vi "CAN loopback test.vi"() -> ()   [LabVIEW 2014]
uses:
  <vilib>/Utility/sysdir.llb/System Directory Type.ctl
  <vilib>/xnet/xnet.llb/XNET Frame CAN.ctl
  <vilib>/xnet/xnet.llb/XNET Frame Type CAN.ctl
  <vilib>/xnet/xnet.llb/XNET Create Session (Frame Input Stream).vi
  <vilib>/xnet/xnet.llb/XNET Create Session (Frame Output Stream).vi
  <vilib>/xnet/xnet.llb/XNET Write (Frame CAN).vi
  <vilib>/xnet/xnet.llb/XNET Read (Frame CAN).vi
  <resource>/objmgr/xnet.rc
panel:
  out "iteration":i32
  out "Frame Passed":bool
  in  "Suspected interface (transmitting)":refnum<k21>="CAN2"
  in  "Termination - set to On, since cables are unterminated":u32(ring)=1 items=["Off", "On"]
  in  "Receiving CAN port (known good module)":refnum<k21>="CAN1"
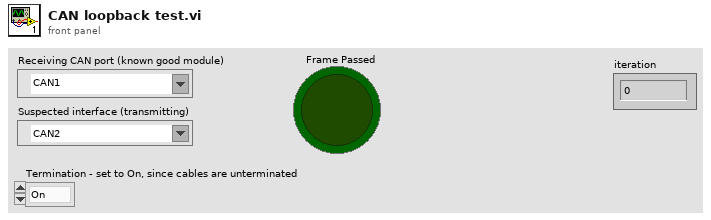
[diagram p1: front panel]
types:
  T1 = typedef "System Directory Type.ctl" = i32
  T2 = enum16{"open", "replace", "create", "open or create", "replace or create", "replace or create with confirmation"}
  T3 = typedef "XNET Frame CAN.ctl" = cluster{"timestamp":timestamp, "payload":u8[], "identifier":u32, "type":T4, "extended?":bool, "echo?":bool}
  T4 = typedef "XNET Frame Type CAN.ctl" = u8
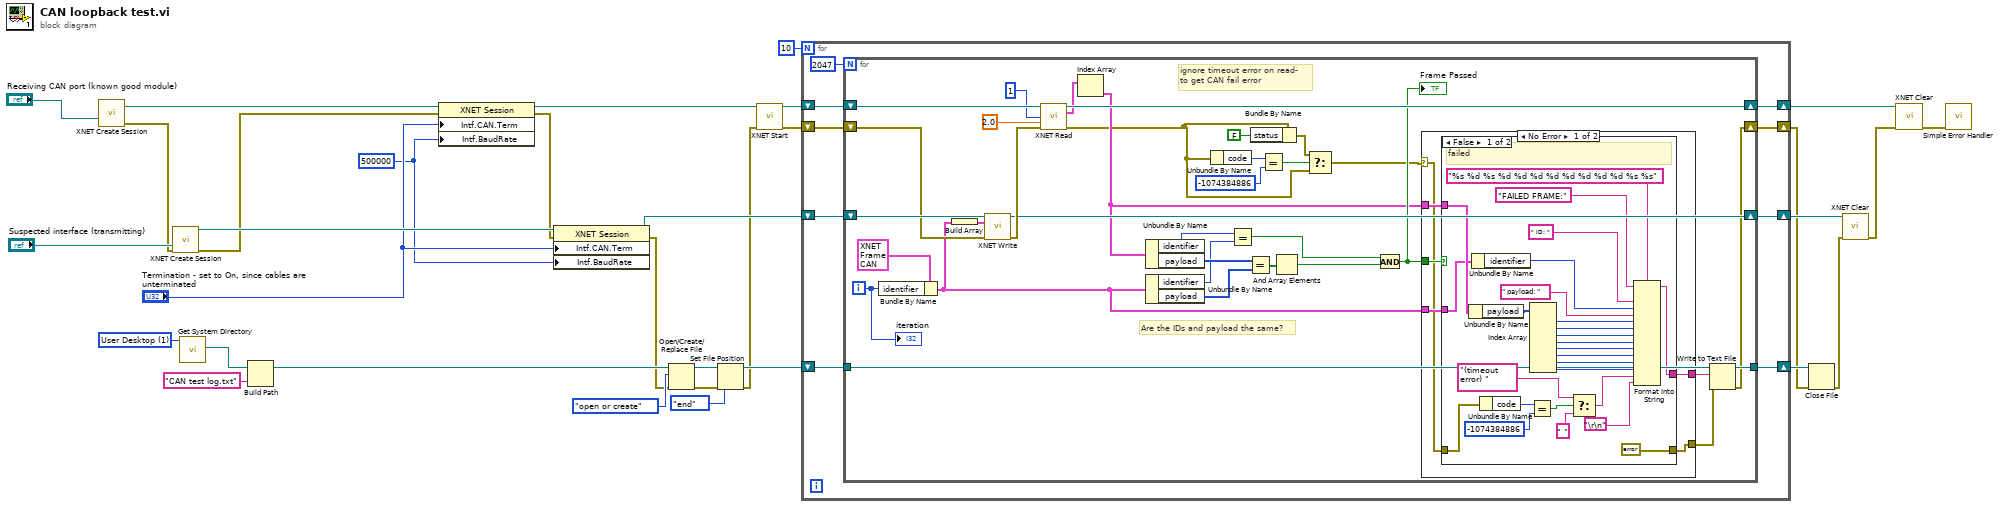
[diagram p0: block diagram]
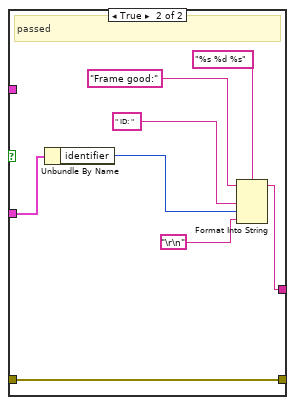
[diagram p2: hidden frame]
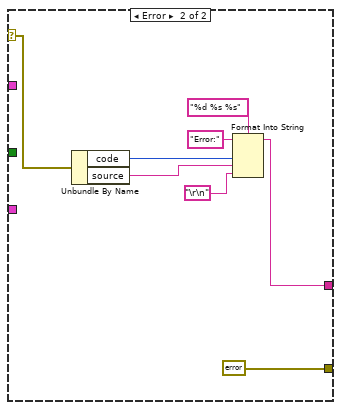
[diagram p3: hidden frame]
diagram:
  w4 = u32 500000 ("Interface:Baud Rate")
  w13 = T1 1 items=["User Home"=0, "User Desktop"=1, "User Documents"=2, "User Application Data"=3, "User Preferences"=4, "User Temporary"=5, "Public Documents"=6, "Public Application Data"=7, "Public Preferences"=8, "Public Cache"=13, "System Core Libraries"=9, "System Installed Libraries"=10, "Application Files"=11, "Boot Volume Root"=12] ("system directory type")
  n1 = call-poly <vilib>:"XNET Create Session.vi"("interface"="Receiving CAN port (known good module)") -> ("session out"=w7:refnum<k21>, "error out"=w28:errorcluster)  [unwired: 2 in, 11 out]
  n2 = call-poly <vilib>:"XNET Create Session.vi"("interface"="Suspected interface (transmitting)", "error in (no error)"=w28) -> ("session out"=w22:refnum<k21>, "error out"=w1:errorcluster)  [unwired: 1 in, 11 out]
  n3 = call <vilib>:"Get System Directory.vi"("system directory type"=w13) -> ("system directory"=w12:path)  [unwired: 10 in]
  n4 = Build Path(base path=w12, name or relative path="CAN test log.txt") -> (appended path=w11:path)
  n5 = property class="XNET Session"(reference=w7, error in=w1, "Intf.CAN.Term"="Termination - set to On, since cables are unterminated", "Intf.BaudRate"=w4) -> (reference out=w6:refnum<k21>, error out=w2:errorcluster)
  n6 = property class="XNET Session"(reference=w22, error in=w2, "Intf.CAN.Term"="Termination - set to On, since cables are unterminated", "Intf.BaudRate"=w4) -> (reference out=w31:refnum<k21>, error out=w9:errorcluster)
  n7 = Open/Create/Replace File(file path (use dialog)=w11, error in=w9, operation (0:open)=T2."open or create") -> (refnum out=w16:refnum<file>, error out=w21:errorcluster)  [unwired: 3 in, 1 out]
  n8 = Set File Position(refnum=w16, from (0:start)=enum16{"start", "end", "current"}."end", error in=w21) -> (refnum out=w15:refnum<file>, error out=w8:errorcluster)  [unwired: 1 in]
  n9 = call <vilib>:"XNET Start.vi"("session in"=w6, "error in (no error)"=w8) -> ("session out"=w27:refnum<k21>, "error out"=w29:errorcluster)  [unwired: 12 in]
  n10 = for {
    N: 10 -> [_]
    shift-right: [w38] -> w26
    shift-left: w31 -> [w41]
    shift-right: [w35] -> w19
    shift-left: w29 -> [w40]
    shift-right: [w37] -> w25
    shift-left: w27 -> [w39]
    shift-right: [w36] -> w20
    shift-left: w15 -> [w34]
    n11 = for {
      N: 2047 ("Numeric Control") -> [_]
      shift-right: [w70] -> w38
      shift-left: w41 -> [w75]
      shift-right: [w49] -> w35
      shift-left: w40 -> [w74]
      shift-right: [w69] -> w37
      shift-left: w39 -> [w72]
      tunnel: w34 -> [w52]
      tunnel: [w53] -> w36
      i -> [w62]
      # "ignore timeout error on read-\nto get CAN fail error"
      # "Are the IDs and payload the same?"
      n12 = Bundle By Name(cluster=T3 {"timestamp"=timestamp(0 s since 1904-01-01), "payload"=[0, 1, 2, 3, 4, 5, 6, 7], "identifier"=0, "type"=0, "extended?"=FALSE, "echo?"=FALSE} ("CAN frame"), "identifier"=w62) -> (w55:T3)
      n13 = Build Array(w55) -> (w61:T3[])
      n14 = call-poly <vilib>:"XNET Write.vi"("session in"=w75, "data"=w61, "error in (no error)"=w74) -> ("session out"=w70:refnum<k21>, "error out"=w73:errorcluster)  [unwired: 11 out]
      n15 = call-poly <vilib>:"XNET Read.vi"("session in"=w72, "number to read (-1)"=1, "timeout (0)"=2.0, "error in (no error)"=w73) -> ("session out"=w69:refnum<k21>, "data"=w63:T3[], "error out"=w44:errorcluster)  [unwired: 8 in, 1 out]
      n16 = Index Array(array=w63) -> (element=w54:T3)  [unwired: 1 in]
      n17 = Unbundle By Name(w54) -> ("identifier"=w58:u32, "payload"=w65:u8[])
      n18 = Unbundle By Name(w55) -> ("identifier"=w59:u32, "payload"=w64:u8[])
      n19 = Unbundle By Name(w44) -> ("code"=w48:i32)
      n20 = Equal?(x=w58, y=w59) -> (x = y?=w57:bool)
      n21 = Equal?(x=w65, y=w64) -> (x = y?=w66:bool[])
      n22 = Bundle By Name(cluster=w44, "status"=FALSE) -> (w42:errorcluster)
      n23 = Equal?(x=w48, y=-1074384886) -> (x = y?=w46:bool)
      n24 = And Array Elements(Boolean array=w66) -> (logical AND=w71:bool)
      n25 = Select(t=w42, s=w46, f=w44) -> (s? t:f=w45:errorcluster)
      n26 = Compound Arithmetic op=AND(w57, w71) -> (w56:bool)
      "Frame Passed" <- w56
      n27 = case shown="No Error" w45 {
        selector: w45 -> [w76 w122]
        tunnel: w56 -> [w81 _]
        tunnel: w55 -> [w80 _]
        tunnel: w54 -> [w79 _]
        tunnel: [w78 w119] -> w51
        tunnel: [w77 errorcluster {"status"=FALSE, "code"=0, "source"=""} ("error IO")] -> w50
        frame No Error {
          n28 = case shown="False" w81 {
            tunnel: w80 -> [w105 w114]
            tunnel: w79 -> [w106 _]
            tunnel: [w91 w111] -> w78
            tunnel: [errorcluster {"status"=FALSE, "code"=0, "source"=""} ("error IO") w108] -> w77
            tunnel: w76 -> [w88 w108]
            frame False {
              # "failed"
              n29 = Unbundle By Name(w106) -> ("payload"=w100:u8[])
              n30 = Unbundle By Name(w105) -> ("identifier"=w104:u32)
              n31 = Unbundle By Name(w88) -> ("code"=w90:i32)
              n32 = Equal?(x=w90, y=-1074384886) -> (x = y?=w86:bool)
              n33 = Index Array(array=w100) -> (element #1=w101:u8, element #2=w99:u8, element #3=w98:u8, element #4=w97:u8, element #5=w96:u8, element #6=w95:u8, element #7=w94:u8, element #8=w93:u8)  [unwired: 8 in]
              n34 = Select(t="(timeout error) " ("initial string"), s=w86, f=" " ("initial string")) -> (s? t:f=w84:string)
              n35 = Format Into String(format string="%s %d %s %d %d %d %d %d %d %d %d %s %s", initial string="FAILED FRAME:", " ID: " ("initial string"), w104, " payload: " ("initial string"), w101, w99, w98, w97, w96, w95, w94, w93, w84, "\r\n") -> (resulting string=w91:string)  [unwired: 1 in, 1 out]
            }
            frame True {
              # "passed"
              n36 = Unbundle By Name(w114) -> ("identifier"=w113:u32)
              n37 = Format Into String(format string="%s %d %s", initial string="Frame good:", " ID: " ("initial string"), w113, "\r\n") -> (resulting string=w111:string)  [unwired: 1 in, 1 out]
            }
          }
        }
        frame Error {
          n38 = Unbundle By Name(w122) -> ("code"=w121:i32, "source"=w120:string)
          n39 = Format Into String(format string="%d %s %s", initial string="Error:", w121, w120, "\r\n") -> (resulting string=w119:string)  [unwired: 1 in, 1 out]
        }
      }
      n40 = Write to Text File(file (use dialog)=w52, text=w51, error in=w50) -> (refnum out=w53:refnum<file>, error out=w49:errorcluster)  [unwired: 1 in, 1 out]
      "iteration" <- w62
    }
  }
  n41 = Close File(refnum=w20, error in=w19) -> (error out=w18:errorcluster)  [unwired: 1 out]
  n42 = call <vilib>:"XNET Clear.vi"("session in"=w26, "error in (no error)"=w18) -> ("error out"=w24:errorcluster)  [unwired: 13 in]
  n43 = call <vilib>:"XNET Clear.vi"("session in"=w25, "error in (no error)"=w24) -> ("error out"=w23:errorcluster)  [unwired: 13 in]
  n44 = call <vilib>:"Simple Error Handler.vi"("error in (no error)"=w23) -> ()  [unwired: 4 in, 5 out]
